vi "Chart[Template].TestLauncher.vi"() -> ()   [LabVIEW 2019, in "Chart[Template].lvclass"]
doc: "JKI State Machine Objects (SMO) 1.0.0.5\nJKI - JKI\nCopyright (c) 2016, JKI"
uses:
  Chart[Template].lvclass
  C:/Users/Patrick/Documents/GitHub/Test (LV2019)/lv-venv/lv.lib/vi.lib/JKI/JKI SMO/SMO/SMO.lvclass
  C:/Users/Patrick/Documents/GitHub/Test (LV2019)/lv-venv/lv.lib/vi.lib/JKI/JKI SMO/SMO.UI/SMO.UI.lvclass
  Typedefs/Dependencies--Cluster.ctl
  vi.lib/JKI/JKI SMO/SMO/SMO.lvclass
  vi.lib/JKI/JKI SMO/SMO/Typedefs/SMOState --Enum.ctl
  vi.lib/JKI/JKI SMO/SMO.UI/SMO.UI.lvclass
panel:
  in  "Send":bool
  out "error out":errorcluster
  in  "Stop":bool
  # "Chart Test Launcher"
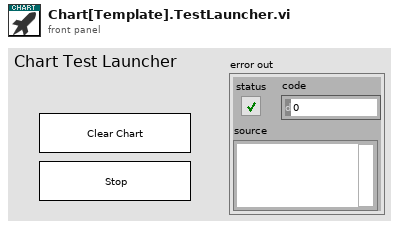
[diagram p1: front panel]
types:
  T1 = typedef "Chart[Template].lvclass/Dependencies--Cluster.ctl" = cluster{"SMO":refnum<class "SMO.lvclass">, "New Value":refnum<user-event>}
  T2 = typedef "SMO.lvclass/Public Events.ctl" = cluster{"Error":refnum<user-event>, "State":refnum<user-event>, "Reserve State":refnum<user-event>}
  T3 = typedef "SMO.UI.lvclass/PublicEvents--Cluster.ctl" = cluster{"UI Hidden":refnum<user-event>, "UI State":refnum<user-event>}
  T4 = typedef "Chart[Template].lvclass/PublicEvents--Cluster.ctl" = cluster{"Chart cleared":refnum<user-event>}
  T5 = typedef "SMO.lvclass/SMOState --Enum.ctl" = enum16{"unknown", "Created", "Started", "Stopped"}
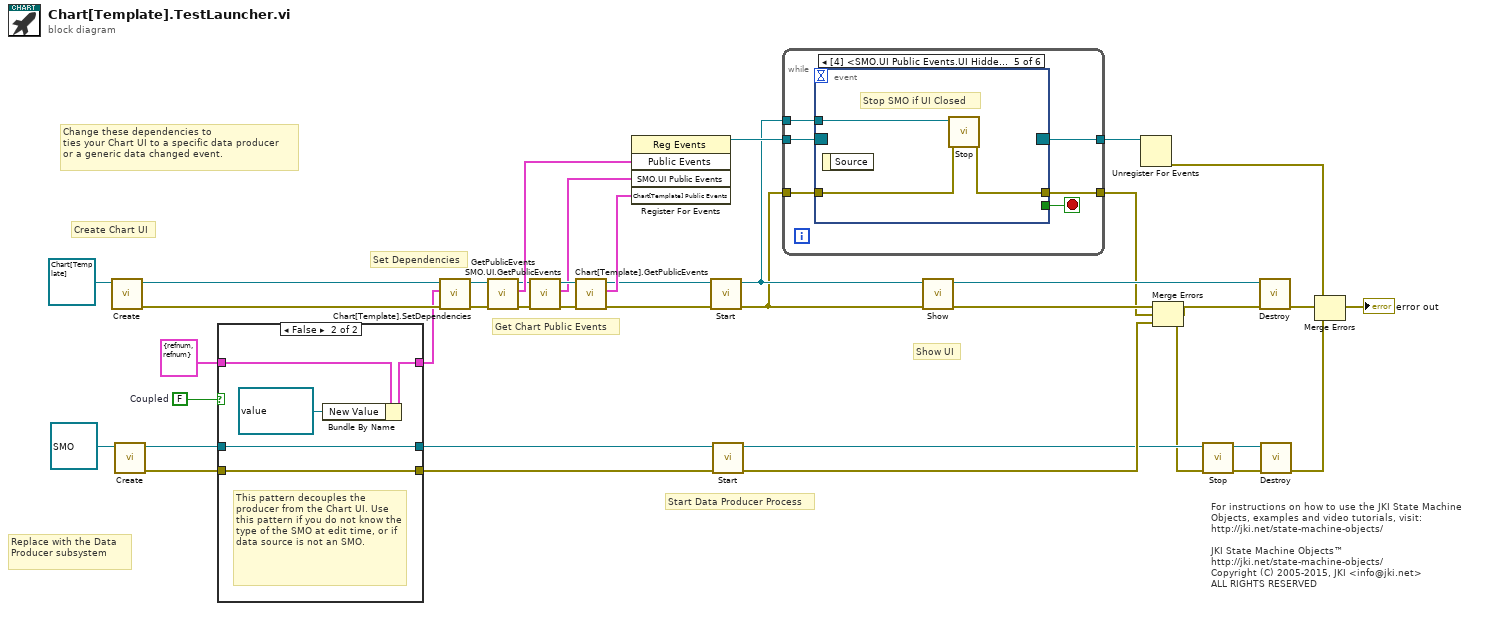
[diagram p0: block diagram]
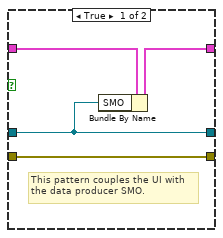
[diagram p2: hidden frame]
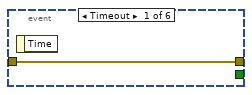
[diagram p3: hidden frame]
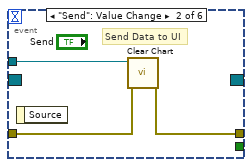
[diagram p4: hidden frame]
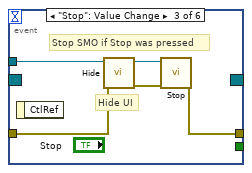
[diagram p5: hidden frame]
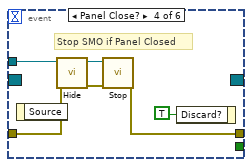
[diagram p6: hidden frame]
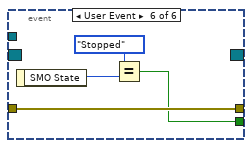
[diagram p7: hidden frame]
diagram:
  w22 = FALSE  # Coupled
  # "Start Data Producer Process"
  # "Set Dependencies"
  # "Create Chart UI"
  # "Replace with the Data Producer subsystem"
  # "Change these dependencies to\nties your Chart UI to a specific data producer\nor a generic data changed event."
  # "Show UI"
  # "For instructions on how to use the JKI State Machine Objects, examples and video tutorials, visit:\nhttp://jki.net/state-machine-objects/\n\nJKI State Machine Objects™\nhttp://jki.net/state-machine-objects/\nCopyright (C) 2005-2015, JKI <info@jki.net>\nALL RIGHTS RESERVED"
  # "Get Chart Public Events"
  n1 = call "Create.vi"("SMO"=refnum<class "Chart[Template].lvclass"> refnum ("Chart[Template]")) -> ("error out"=w31:errorcluster, "SMO out"=w32:refnum<class "Chart[Template].lvclass">)  [unwired: 8 in, 1 out]
  n2 = call "Create.vi"("SMO"=refnum<class "SMO.lvclass"> refnum) -> ("error out"=w18:errorcluster, "SMO out"=w21:refnum<class "SMO.lvclass">)  [unwired: 8 in, 1 out]
  n3 = case shown="False" w22 {
    tunnel: T1 {"SMO"=refnum, "New Value"=refnum} ("Dependencies") -> [w42 w47]
    tunnel: [w41 w46] -> w23
    tunnel: w21 -> [w40 w44]
    tunnel: [w40 w44] -> w20
    tunnel: [w39 w43] -> w19
    tunnel: w18 -> [w39 w43]
    frame True {
      # "This pattern couples the UI with\nthe data producer SMO."
      n4 = Bundle By Name(cluster=w42, "SMO"=w40) -> (w41:T1)
    }
    frame False {
      # "This pattern decouples the producer from the Chart UI. Use this pattern if you do not know the type of the SMO at edit time, or if data source is not an SMO."
      n5 = Bundle By Name(cluster=w47, "New Value"=refnum<user-event> refnum) -> (w46:T1)
    }
  }
  n6 = call "Chart[Template].SetDependencies.vi"("error in (no error)"=w31, "Dependencies"=w23, "Chart[Template]"=w32) -> ("error out"=w5:errorcluster, "Chart[Template] out"=w17:refnum<class "Chart[Template].lvclass">)  [unwired: 7 in]
  n7 = call "GetPublicEvents.vi"("error in (no error)"=w5, "SMO"=w17) -> ("error out"=w12:errorcluster, "Public Events"=w16:T2, "SMO out"=w14:refnum<class "Chart[Template].lvclass">)  [unwired: 7 in]
  n8 = call "SMO.UI.GetPublicEvents.vi"("error in (no error)"=w12, "SMO.UI"=w14) -> ("error out"=w11:errorcluster, "SMO.UI Public Events"=w10:T3, "SMO.UI out"=w13:refnum<class "Chart[Template].lvclass">)  [unwired: 7 in]
  n9 = call "Chart[Template].GetPublicEvents.vi"("error in (no error)"=w11, "Chart[Template]"=w13) -> ("error out"=w6:errorcluster, "Chart[Template] Public Events"=w15:T4, "Chart[Template] out"=w7:refnum<class "Chart[Template].lvclass">)  [unwired: 7 in]
  n10 = register-events(w16, w10, w15) -> (reference out=w9:refnum<event-registration>)  [unwired: 2 in, 1 out]
  n11 = call "Start.vi"("error in (no error)"=w6, "SMO"=w7) -> ("error out"=w2:errorcluster, "SMO out"=w8:refnum<class "Chart[Template].lvclass">)  [unwired: 8 in]
  n12 = call "Start.vi"("error in (no error)"=w19, "SMO"=w20) -> ("error out"=w29:errorcluster, "SMO out"=w28:refnum<class "SMO.lvclass">)  [unwired: 8 in]
  n13 = while {
    tunnel: w9 -> [w52]
    tunnel: [w51] -> w38
    tunnel: w8 -> [w50]
    tunnel: w2 -> [w49]
    tunnel: [w48] -> w1
    stop <- w53 stop-if-true
    n14 = event shown="[4] <SMO.UI Public Events.UI Hidden>: User Event" {
      selector: w52 -> [_ _ _ _ _ _]
      dyn-events: [_ _ _ _ _ _] -> w51
      timeout: _ -> [_ _ _ _ _ _]
      tunnel: [_ _ _ _ _ w72] -> w53
      tunnel: w50 -> [_ w57 w61 w66 w70 _]
      tunnel: [w54 w55 w62 w68 w71 w75] -> w48
      tunnel: w49 -> [w54 w56 w59 w64 w69 w75]
      event Timeout {
        n15 = event-data() -> ()  [unwired: 1 in, 1 out]
      }
      event "Send": Value Change {
        # "Send Data to UI"
        n16 = event-data() -> ()  [unwired: 1 in, 1 out]
        n17 = call "Clear Chart.vi"("error in (no error)"=w56, "Chart[Template]"=w57) -> ("error out"=w55:errorcluster)  [unwired: 8 in, 1 out]
      }
      event "Stop": Value Change {
        # "Hide UI"
        # "Stop SMO if Stop was pressed"
        n18 = event-data() -> ()  [unwired: 1 in, 1 out]
        n19 = call "Hide.vi"("error in (no error)"=w59, "SMO.UI"=w61) -> ("error out"=w58:errorcluster, "SMO.UI out"=w60:refnum<class "Chart[Template].lvclass">)  [unwired: 8 in]
        n20 = call "Stop.vi"("error in (no error)"=w58, "SMO"=w60) -> ("error out"=w62:errorcluster)  [unwired: 8 in, 1 out]
      }
      event Panel Close? {
        # "Stop SMO if Panel Closed"
        n21 = event-data() -> ()  [unwired: 1 in, 1 out]
        n22 = call "Hide.vi"("error in (no error)"=w64, "SMO.UI"=w66) -> ("error out"=w63:errorcluster, "SMO.UI out"=w65:refnum<class "Chart[Template].lvclass">)  [unwired: 8 in]
        n23 = call "Stop.vi"("error in (no error)"=w63, "SMO"=w65) -> ("error out"=w68:errorcluster)  [unwired: 8 in, 1 out]
        n24 = event-data("Discard?"=TRUE ("OK")) -> ()  [unwired: 1 in, 1 out]
      }
      event User Event {
        # "Stop SMO if UI Closed"
        n25 = event-data() -> ()  [unwired: 1 in, 1 out]
        n26 = call "Stop.vi"("error in (no error)"=w69, "SMO"=w70) -> ("error out"=w71:errorcluster)  [unwired: 8 in, 1 out]
      }
      event User Event {
        n27 = event-data() -> ("SMO State"=w74:T5)  [unwired: 1 in]
        n28 = Equal?(x=SMOState_--Enum."Stopped", y=w74) -> (x = y?=w72:bool)
      }
    }
  }
  n29 = call "Show.vi"("error in (no error)"=w2, "SMO.UI"=w8) -> ("error out"=w33:errorcluster, "SMO.UI out"=w4:refnum<class "Chart[Template].lvclass">)  [unwired: 8 in]
  n30 = Unregister For Events(event registration refnum=w38) -> (error out=w37:errorcluster)  [unwired: 1 in]
  n31 = Merge Errors(w33, w1, w29) -> (w3:errorcluster)
  n32 = call "Stop.vi"("error in (no error)"=w3, "SMO"=w28) -> ("error out"=w27:errorcluster, "SMO out"=w26:refnum<class "SMO.lvclass">)  [unwired: 8 in]
  n33 = call "Destroy.vi"("error in (no error)"=w3, "SMO"=w4) -> ("error out"=w35:errorcluster)  [unwired: 9 in]
  n34 = call "Destroy.vi"("error in (no error)"=w27, "SMO"=w26) -> ("error out"=w25:errorcluster)  [unwired: 9 in]
  n35 = Merge Errors(w37, w35, w25) -> (→"error out":errorcluster)
